vi "Game Piece State to Shoulder and Extender Encoder Positions.vi"(5 "Arm Offset (Inches)":dbl, 7 "Wrist Offset (Inches)":dbl, 8 "Wrist Enc Position":dbl, 10 "Z (Inches)":dbl, 11 "X (Inches)":dbl) -> (1 "Target Extender Enc Pos":dbl, 3 "Target Shoulder Enc Pos":dbl)   [LabVIEW 2023]
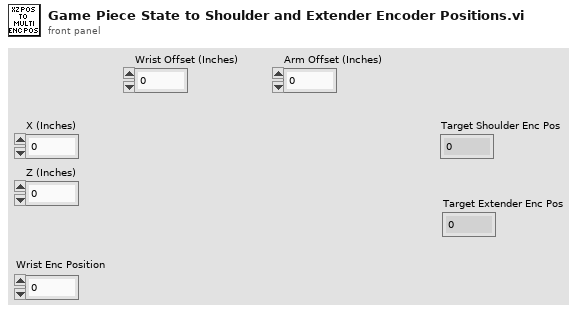
[diagram p1: front panel]
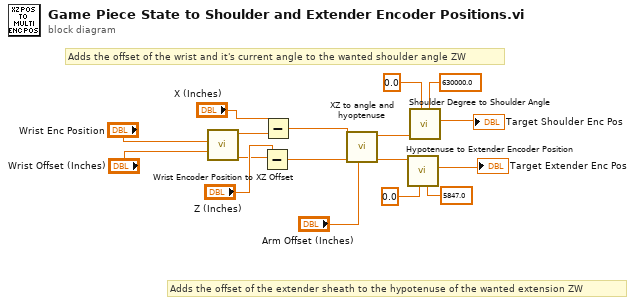
[diagram p0: block diagram]
diagram:
  # "Adds the offset of the extender sheath to the hypotenuse of the wanted extension ZW"
  # "Adds the offset of the wrist and it's current angle to the wanted shoulder angle ZW"
  n1 = call "Wrist Encoder Position to XZ Offset.vi"("Wrist Offset (Inches)"="Wrist Offset (Inches)", "Wrist Enc Pos"="Wrist Enc Position") -> ("Wrist Z"=w11:dbl, "Wrist X"=w14:dbl)  [unwired: 8 in]
  n2 = Subtract(x="Z (Inches)", y=w11) -> (x-y=w10:dbl)
  n3 = Subtract(x="X (Inches)", y=w14) -> (x-y=w13:dbl)
  n4 = call "XZ to angle and hyoptenuse.vi"("Arm Offset (Inches)"="Arm Offset (Inches)", "Z"=w10, "X"=w13) -> ("Hypotenuse (Inches)"=w5:dbl, "Angle (degrees)"=w9:dbl)  [unwired: 7 in]
  n5 = call "Hypotenuse to Extender Encoder Position.vi"("Extender Enc Pos at 12 inches"=5847.0, "Min Extender Enc Pos"=0.0, "Wanted Extension (Inches)"=w5) -> ("Target Extender Enc Pos"=→"Target Extender Enc Pos":dbl)  [unwired: 8 in]
  n6 = call "Shoulder Degree to Shoulder Angle.vi"("Level Shoulder Enc Pos"=630000.0, "Min Shoulder Enc Pos"=0.0, "Wanted Shoulder Angle (Degrees)"=w9) -> ("Target Shoulder Enc Pos"=→"Target Shoulder Enc Pos":dbl)  [unwired: 8 in]
